vi "STM Read Meta.vi"(8 "error in":errorcluster, 10 "timeout ms (25000)":i32=25000, 11 "connection ID":refnum<k5>) -> (0 "error out":errorcluster, 1 "Meta data":T1[](array[typedef]), 3 "connection ID out":refnum<k5>)   [LabVIEW 2014, in "QwaveSys Raspberry Pi Library.lvlib"]
doc: "This VI reads the meta data information from a remote computer. Use this VI to retrieve the variable names and types that a remote computer exports.\n\nThis VI parses the data and returns a cluster containing the meta data information."
uses:
  _SubVIs/TypeDefs/stm_MetaElement.ctl
  QwaveSys Raspberry Pi Library.lvlib
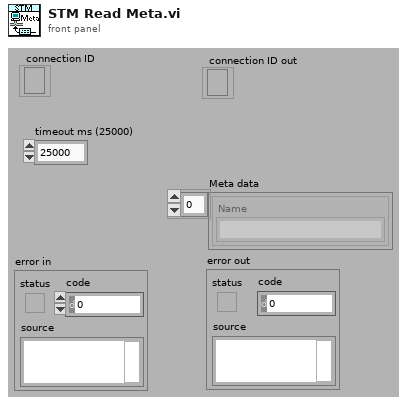
[diagram p1: front panel]
types:
  T1 = typedef "QwaveSys Raspberry Pi Library.lvlib/stm_MetaElement.ctl" = cluster{"Name":string}
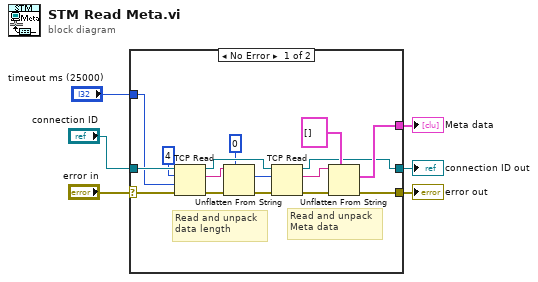
[diagram p0: block diagram]
diagram:
  n1 = case shown="No Error" "error in" {
    selector: "error in" -> [w8 w23]
    tunnel: [w22 _] -> w6
    tunnel: [w21 w23] -> w5
    tunnel: "connection ID" -> [w19 w24]
    tunnel: [w14 w24] -> w3
    tunnel: "timeout ms (25000)" -> [w7 _]
    frame No Error {
      # "Read and unpack\nMeta data"
      # "Read and unpack\ndata length"
      n2 = TCP Read(connection ID=w19, bytes to read=4, error in (no error)=w8, 9:w7) -> (connection ID out=w17:refnum<k5>, data out=w13:string, error out=w9:errorcluster)  [unwired: 1 out]
      n3 = Unflatten From String(type=0 ("bytes to read"), binary string=w13, error in (no error)=w9) -> (value=w10:i32, error out=w11:errorcluster)  [unwired: 3 out]
      n4 = TCP Read(connection ID=w17, bytes to read=w10, error in (no error)=w11) -> (connection ID out=w14:refnum<k5>, data out=w16:string, error out=w15:errorcluster)  [unwired: 2 out]
      n5 = Unflatten From String(type=T1[] [] ("Meta data"), binary string=w16, error in (no error)=w15) -> (value=w22:T1[], error out=w21:errorcluster)  [unwired: 3 out]
    }
    frame Error {
    }
  }
  "Meta data" <- w6
  "error out" <- w5
  "connection ID out" <- w3
